vi "Start Sync.vi"(8 "error in (no error)":errorcluster, 10 "current time":timestamp, 11 "gRPC Server in":refnum<class "HVC.lvclass">) -> (0 "error out":errorcluster, 3 "gRPC Server out":refnum<class "HVC.lvclass">)   [LabVIEW 2019, in "HVC.lvlib" / "HVC.lvclass"]
uses:
  HVC.lvclass
  HVC.lvclass/HVC.ctl
  RPC Messages/measurementservice_QueryResponse/measurementservice_QueryResponse_Data.ctl
  RPC Messages/measurementservice_ErrorOut/measurementservice_ErrorOut_Data.ctl
  RPC Messages/measurementservice_DMMConfigRequest/measurementservice_DMMConfigRequest_Data.ctl
  RPC Messages/measurementservice_DMMConfigResponse/measurementservice_DMMConfigResponse_Data.ctl
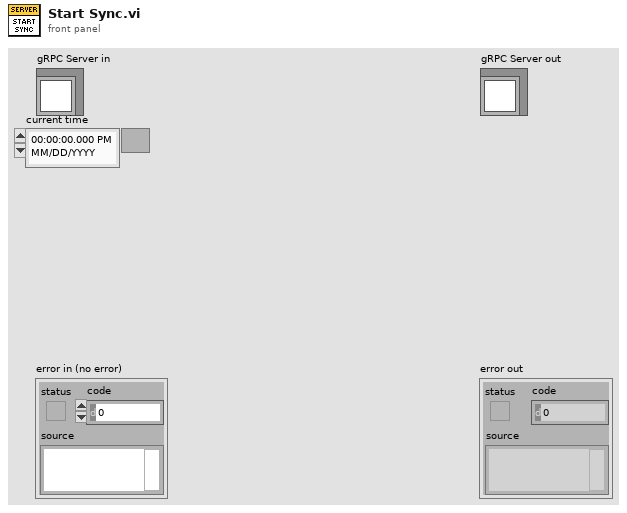
[diagram p1: front panel]
types:
  T1 = typedef "HVC.lvlib/HVC.lvclass/measurementservice_DMMConfigRequest_Data.ctl" = cluster{"DMMFunction":i32, "DMMResolution":sgl, "DMMRange":sgl, "DMMSampleCount":i32, "DMMApertureTimeUnit":i32, "DMMApertureTime":sgl, "DMMNumberofAverages":i32, "DMMAutoZero":i32, "DMMADCCalibration":i32, "DMMSettleTime":sgl, "error":T2}
  T2 = typedef "HVC.lvlib/HVC.lvclass/measurementservice_ErrorOut_Data.ctl" = cluster{"errCode":i32, "errMessage":string}
  T3 = cluster{"measurementservice_DMMConfigRequest_Data":T1}
  T4 = typedef "HVC.lvlib/HVC.lvclass/measurementservice_QueryResponse_Data.ctl" = cluster{"message":string, "status":i32}
  T5 = typedef "HVC.lvlib/HVC.lvclass/measurementservice_DMMConfigResponse_Data.ctl" = cluster{"DMMFunction":i32, "DMMResolution":sgl, "DMMRange":sgl, "DMMSampleCount":i32, "DMMApertureTimeUnit":i32, "DMMApertureTime":sgl, "DMMNumberofAverages":i32, "DMMAutoZero":i32, "DMMADCCalibration":i32, "DMMSettleTime":sgl, "error":T2}
  T6 = typedef "HVC.lvlib/HVC.lvclass/Server gRPC UEs.ctl" = cluster{"Invoke gRPC UE":refnum<user-event>, "Query gRPC UE":refnum<user-event>, "Register gRPC UE":refnum<user-event>, "ConfigureDMM gRPC UE":refnum<user-event>, "PerformDMMVoltageMeasurement gRPC UE":refnum<user-event>}
  T7 = typedef "HVC.lvlib/gprc-lvsupport.lvlib/grpcId.ctl" = u64
  T8 = typedef "HVC.lvlib/HVC.lvclass/measurementservice_QueryRequest_Data.ctl" = cluster{"query":string}
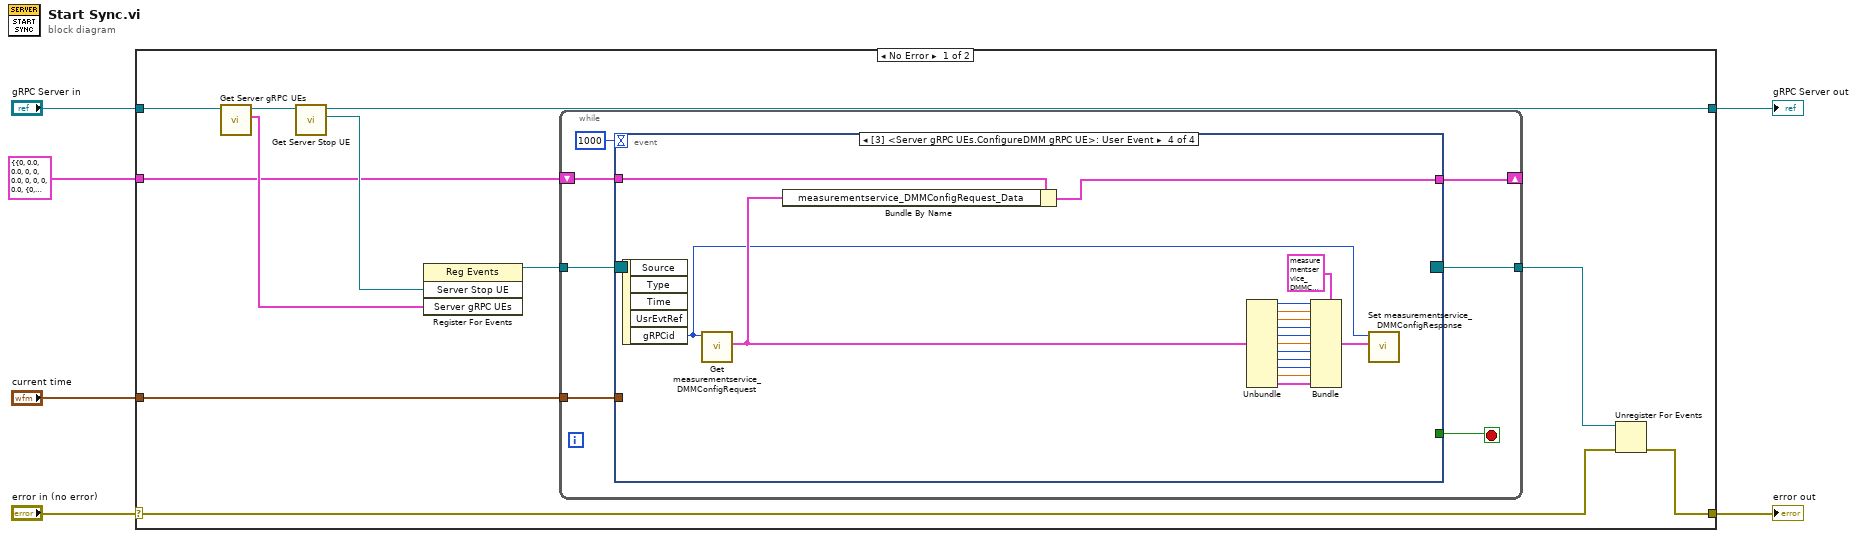
[diagram p0: block diagram]
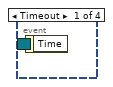
[diagram p2: hidden frame]
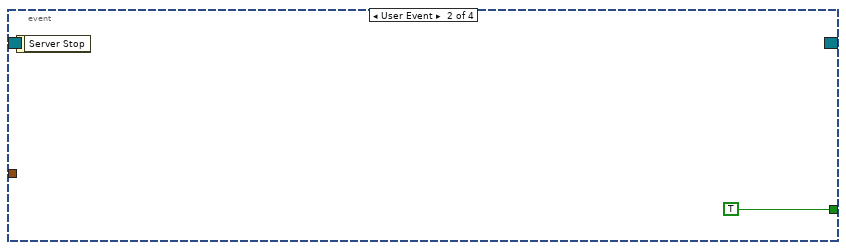
[diagram p3: hidden frame]
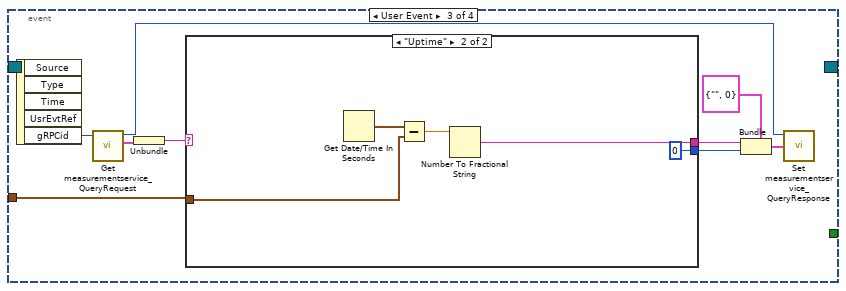
[diagram p4: hidden frame]
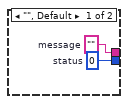
[diagram p5: hidden frame]
diagram:
  n1 = case shown="No Error" "error in (no error)" {
    selector: "error in (no error)" -> [w10 w60]
    tunnel: [w9 w60] -> w5
    tunnel: [w13 w59] -> w3
    tunnel: "gRPC Server in" -> [w17 w59]
    tunnel: "current time" -> [w8 _]
    tunnel: T3 {"measurementservice_DMMConfigRequest_Data"={"DMMFunction"=0, "DMMResolution"=0.0, "DMMRange"=0.0, "DMMSampleCount"=0, "DMMApertureTimeUnit"=0, "DMMApertureTime"=0.0, "DMMNumberofAverages"=0, "DMMAutoZero"=0, "DMMADCCalibration"=0, "DMMSettleTime"=0.0, "error"={"errCode"=0, "errMessage"=""}}} -> [w7 _]
    frame No Error {
      n2 = call "Get Server gRPC UEs.vi"("OOP Server in"=w17) -> ("Server gRPC UEs"=w14:T6, "OOP Server out"=w16:refnum<class "HVC.lvclass">)  [unwired: 9 in]
      n3 = call "Get Server Stop UE.vi"("OOP Server in"=w16) -> ("Server Stop UE"=w15:refnum<user-event>, "OOP Server out"=w13:refnum<class "HVC.lvclass">)  [unwired: 9 in]
      n4 = register-events(w15, w14) -> (reference out=w12:refnum<event-registration>)  [unwired: 2 in, 1 out]
      n5 = while {
        tunnel: w12 -> [w24]
        tunnel: [w22] -> w11
        tunnel: w8 -> [w20]
        shift-right: [w18] -> _
        shift-left: w7 -> [w19]
        stop <- w23 stop-if-true
        n6 = event "RPC Methods Event Structure" shown="[3] <Server gRPC UEs.ConfigureDMM gRPC UE>: User Event" {
          selector: w24 -> [_ _ _ _]
          dyn-events: [_ _ _ _] -> w22
          timeout: 1000 -> [_ _ _ _]
          tunnel: [_ TRUE _ _] -> w23
          tunnel: w20 -> [_ _ w26 _]
          tunnel: [_ _ _ w57] -> w18
          tunnel: w19 -> [_ _ _ w58]
          event Timeout {
            n7 = event-data() -> ()  [unwired: 1 in, 1 out]
          }
          event User Event {
            n8 = event-data() -> ()  [unwired: 1 in, 1 out]
          }
          event User Event {
            n9 = event-data() -> ("gRPCid"=w34:T7)  [unwired: 1 in, 4 out]
            n10 = call "Get measurementservice_QueryRequest.vi"("gRPCid"=w34) -> ("Message Data"=w33:T8, "gRPCid out"=w32:T7)  [unwired: 8 in, 1 out]
            n11 = Unbundle(w33) -> ("query"=w29:string)
            n12 = case shown="\"Uptime\"" w29 {
              tunnel: [w36 0 ("status")] -> w28
              tunnel: [w35 w38] -> w27
              tunnel: w26 -> [_ w40]
              frame "", Default {
                w35 = ""  # message
                w36 = 0  # status
              }
              frame "Uptime" {
                n13 = Get Date/Time In Seconds() -> (seconds since 1Jan1904=w41:timestamp)
                n14 = Subtract(x=w41, y=w40) -> (x-y=w39:dbl)
                n15 = Number To Fractional String(number=w39) -> (F-format string=w38:string)  [unwired: 3 in]
              }
            }
            n16 = Bundle(cluster=T4 {"message"="", "status"=0} ("measurementservice_QueryResponse_Data"), "message"=w27, "status"=w28) -> (w30:T4)
            n17 = call "Set measurementservice_QueryResponse.vi"("Message Data"=w30, "gRPCid"=w32) -> ()  [unwired: 9 in, 1 out]
          }
          event User Event {
            n18 = event-data() -> ("gRPCid"=w53:T7)  [unwired: 1 in, 4 out]
            n19 = call "Get measurementservice_DMMConfigRequest.vi"("gRPCid"=w53) -> ("Message Data"=w54:T1)  [unwired: 8 in, 2 out]
            n20 = Bundle By Name(cluster=w58, "measurementservice_DMMConfigRequest_Data"=w54) -> (w57:T3)
            n21 = Unbundle(w54) -> ("DMMFunction"=w52:i32, "DMMResolution"=w51:sgl, "DMMRange"=w50:sgl, "DMMSampleCount"=w49:i32, "DMMApertureTimeUnit"=w48:i32, "DMMApertureTime"=w47:sgl, "DMMNumberofAverages"=w46:i32, "DMMAutoZero"=w45:i32, "DMMADCCalibration"=w44:i32, "DMMSettleTime"=w43:sgl, "error"=w42:T2)
            n22 = Bundle(cluster=T5 {"DMMFunction"=0, "DMMResolution"=0.0, "DMMRange"=0.0, "DMMSampleCount"=0, "DMMApertureTimeUnit"=0, "DMMApertureTime"=0.0, "DMMNumberofAverages"=0, "DMMAutoZero"=0, "DMMADCCalibration"=0, "DMMSettleTime"=0.0, "error"={"errCode"=0, "errMessage"=""}} ("measurementservice_DMMConfigResponse_Data"), "DMMFunction"=w52, "DMMResolution"=w51, "DMMRange"=w50, "DMMSampleCount"=w49, "DMMApertureTimeUnit"=w48, "DMMApertureTime"=w47, "DMMNumberofAverages"=w46, "DMMAutoZero"=w45, "DMMADCCalibration"=w44, "DMMSettleTime"=w43, "error"=w42) -> (w55:T5)
            n23 = call "Set measurementservice_DMMConfigResponse.vi"("Message Data"=w55, "gRPCid"=w53) -> ()  [unwired: 9 in, 1 out]
          }
        }
      }
      n24 = Unregister For Events(event registration refnum=w11, error in=w10) -> (error out=w9:errorcluster)
    }
    frame Error {
    }
  }
  "error out" <- w5
  "gRPC Server out" <- w3
